vi "CreateTablStruct_01.vi"() -> (0 "Array":T3(array[cluster]))   [LabVIEW 2010]
uses:
  <vilib>/addons/database/Auxilliary.llb/DB Tools Column Info.ctl
  <vilib>/addons/database/Auxilliary.llb/DB Tools DataTypes.ctl
  <vilib>/addons/database/NI_Database_API.lvlib
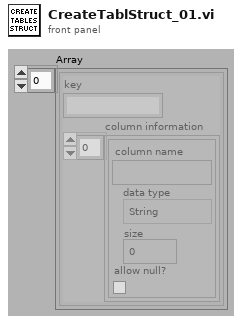
[diagram p1: front panel]
types:
  T1 = typedef "NI_Database_API.lvlib/DB Tools Column Info.ctl" = cluster{"column name":string, "data type":T2, "size":i32, "allow null?":bool}
  T2 = typedef "NI_Database_API.lvlib/DB Tools DataTypes.ctl" = enum16{"String", "Long (I32)", "Single (SGL)", "Double (DBL)", "Date/Time", "Binary"}
  T3 = cluster{"key":string, "column information":T1[]}[]
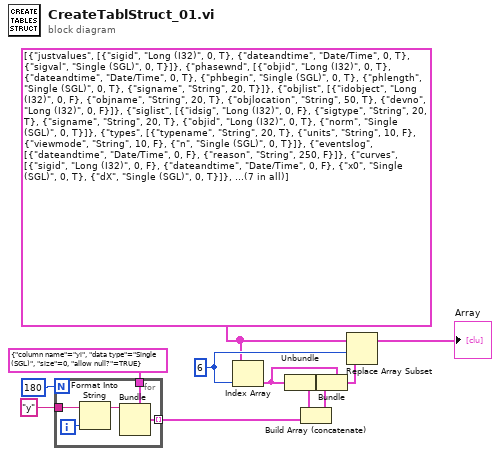
[diagram p0: block diagram]
diagram:
  w8 = 6 ("index")
  w6 = T3 [{"key"="justvalues", "column information"=[{"column name"="sigid", "data type"=enum."Long (I32)", "size"=0, "allow null?"=TRUE}, {"column name"="dateandtime", "data type"=enum."Date/Time", "size"=0, "allow null?"=TRUE}, {"column name"="sigval", "data type"=enum."Single (SGL)", "size"=0, "allow null?"=TRUE}]}, {"key"="phasewnd", "column information"=[{"column name"="objid", "data type"=enum."Long (I32)", "size"=0, "allow null?"=TRUE}, {"column name"="dateandtime", "data type"=enum."Date/Time", "size"=0, "allow null?"=TRUE}, {"column name"="phbegin", "data type"=enum."Single (SGL)", "size"=0, "allow null?"=TRUE}, {"column name"="phlength", "data type"=enum."Single (SGL)", "size"=0, "allow null?"=TRUE}, {"column name"="signame", "data type"=enum."String", "size"=20, "allow null?"=TRUE}]}, {"key"="objlist", "column information"=[{"column name"="idobject", "data type"=enum."Long (I32)", "size"=0, "allow null?"=FALSE}, {"column name"="objname", "data type"=enum."String", "size"=20, "allow null?"=TRUE}, {"column name"="objlocation", "data type"=enum."String", "size"=50, "allow null?"=TRUE}, {"column name"="devno", "data type"=enum."Long (I32)", "size"=0, "allow null?"=FALSE}]}, {"key"="siglist", "column information"=[{"column name"="idsig", "data type"=enum."Long (I32)", "size"=0, "allow null?"=FALSE}, {"column name"="sigtype", "data type"=enum."String", "size"=20, "allow null?"=TRUE}, {"column name"="signame", "data type"=enum."String", "size"=20, "allow null?"=TRUE}, {"column name"="objid", "data type"=enum."Long (I32)", "size"=0, "allow null?"=TRUE}, {"column name"="norm", "data type"=enum."Single (SGL)", "size"=0, "allow null?"=TRUE}]}, {"key"="types", "column information"=[{"column name"="typename", "data type"=enum."String", "size"=20, "allow null?"=TRUE}, {"column name"="units", "data type"=enum."String", "size"=10, "allow null?"=FALSE}, {"column name"="viewmode", "data type"=enum."String", "size"=10, "allow null?"=FALSE}, {"column name"="n", "data type"=enum."Single (SGL)", "size"=0, "allow null?"=TRUE}]}, {"key"="eventslog", "column information"=[{"column name"="dateandtime", "data type"=enum."Date/Time", "size"=0, "allow null?"=FALSE}, {"column name"="reason", "data type"=enum."String", "size"=250, "allow null?"=FALSE}]}, {"key"="curves", "column information"=[{"column name"="sigid", "data type"=enum."Long (I32)", "size"=0, "allow null?"=FALSE}, {"column name"="dateandtime", "data type"=enum."Date/Time", "size"=0, "allow null?"=FALSE}, {"column name"="x0", "data type"=enum."Single (SGL)", "size"=0, "allow null?"=TRUE}, {"column name"="dX", "data type"=enum."Single (SGL)", "size"=0, "allow null?"=TRUE}]}]
  n1 = for {
    N: 180 -> [_]
    tunnel: T1 {"column name"="yi", "data type"=enum."Single (SGL)", "size"=0, "allow null?"=TRUE} ("column information") -> [w16]
    tunnel: [w15] -> w2 mode=indexing
    tunnel: "y" ("column name") -> [w12]
    i -> [w13]
    n2 = Format Into String(initial string=w12, w13) -> (resulting string=w14:string)  [unwired: 2 in, 1 out]
    n3 = Bundle(cluster=w16, "column name"=w14) -> (w15:T1)  [unwired: 3 in]
  }
  n4 = Index Array(array=w6, index=w8) -> (element=w4:cluster{"key":string, "column information":T1[]})
  n5 = Unbundle(w4) -> ("column information"=w3:T1[])  [unwired: 1 out]
  n6 = Build Array (concatenate)(w3, w2) -> (w5:T1[])
  n7 = Bundle(cluster=w4, "column information"=w5) -> (w7:cluster{"key":string, "column information":T1[]})  [unwired: 1 in]
  n8 = Replace Array Subset(array=w6, new element=w7, index=w8) -> (→"Array":T3)
